vi "meth.ExecScript.vi"(0 "GLue in":refnum<class "class.GLue.lvclass">, 2 "Script":string, 5 "Argument":variant, 11 "error in":errorcluster, 12 "Name":string, 14 "ms timeout (-1)":i32=-1) -> (4 "GLue out":refnum<class "class.GLue.lvclass">, 6 "Return":variant, 15 "error out":errorcluster)   [LabVIEW 2014, in "GLue.lvlib" / "class.GLue.lvclass"]
uses:
  class.GLue.lvclass
  class.GLue.lvclass/class.GLue.ctl
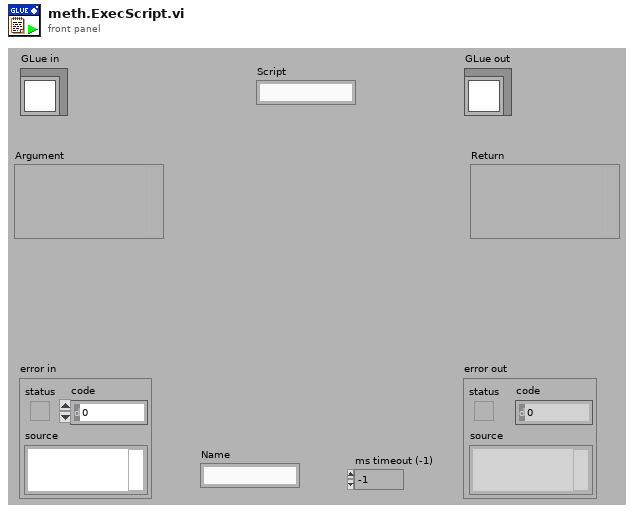
[diagram p1: front panel]
types:
  T1 = typedef "Semaphore RefNum" = refnum<k1>
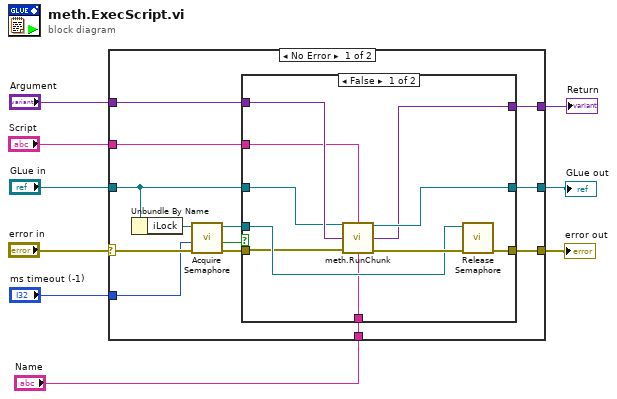
[diagram p0: block diagram]
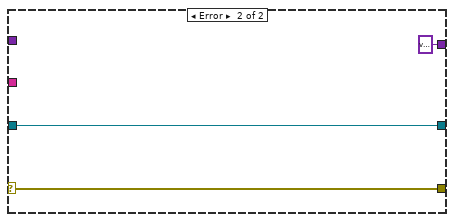
[diagram p3: hidden frame]
diagram:
  n1 = case shown="No Error" "error in" {
    selector: "error in" -> [w18 w38]
    tunnel: [w21 w38] -> w8
    tunnel: [w20 w37] -> w6
    tunnel: "GLue in" -> [w19 w37]
    tunnel: "Script" -> [w22 _]
    tunnel: "ms timeout (-1)" -> [w15 _]
    tunnel: "Argument" -> [w12 _]
    tunnel: [w11 variant ("Data out")] -> w2
    tunnel: "Name" -> [w10 _]
    frame No Error {
      n2 = Unbundle By Name(w19) -> ("iLock"=w16:T1)
      n3 = call <vilib>:"Acquire Semaphore.vi"("error in (no error)"=w18, "ms timeout (-1)"=w15, "semaphore"=w16) -> ("error out"=w17:errorcluster, "timed out"=w14:bool, "semaphore out"=w13:T1)  [unwired: 2 in]
      n4 = case shown="False" w14 {
        tunnel: w22 -> [w24 _]
        tunnel: [w31 w34] -> w21
        tunnel: [w32 w35] -> w20
        tunnel: w19 -> [w26 w35]
        tunnel: w17 -> [w25 w34]
        tunnel: w13 -> [w29 _]
        tunnel: w12 -> [w28 _]
        tunnel: [w27 variant ("Data out")] -> w11
        tunnel: w10 -> [w23 _]
        frame False {
          n5 = call "meth.RunChunk.vi"("GLue in"=w26, "Script"=w24, "Data in"=w28, "error in"=w25, "Name"=w23) -> ("GLue out"=w32:refnum<class "class.GLue.lvclass">, "Data out"=w27:variant, "error out"=w30:errorcluster)  [unwired: 8 in]
          n6 = call <vilib>:"Release Semaphore.vi"("error in (no error)"=w30, "semaphore"=w29) -> ("error out"=w31:errorcluster)  [unwired: 4 in, 1 out]
        }
        frame True {
        }
      }
    }
    frame Error {
    }
  }
  "error out" <- w8
  "GLue out" <- w6
  "Return" <- w2
